vi "PH_PP_CurrentMeas.PC read PA and FR.vi"(0 "i ref in":refnum<vi>, 5 "error in (no error)":errorcluster) -> (14 "i ref out":refnum<vi>, 19 "error out":errorcluster)   [LabVIEW 2014, in "PH_PP_CurrentMeas.lvlib"]
doc: "This VI reads the data from RT client 3 (PA and FR) and sets the GUI elements (if chosen)."
uses:
  PH_PP_CurrentMeas.lvlib
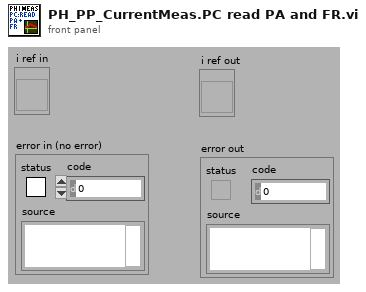
[diagram p1: front panel]
types:
  T1 = typedef "PH_PP_CurrentMeas.lvlib/PH_PP_CurrentMeas.i attribute.ctl" = cluster{"Status":cluster{"GUI Ref Hardware Feedback":refnum<vi>, "Tab Control":refnum<vi>}, "PU 1":cluster{"Instance":string, "Status":T2, "Ref Status ":refnum<vi>, "Data":waveform(dbl)[], "Ref Data":refnum<vi>}, "PU 2":cluster{"Instance":string, "Status":T2, "Ref Status ":refnum<vi>, "Data":waveform(dbl)[], "Ref Data":refnum<vi>}, "PU 3":cluster{"Instance":string, "Status":T2, "Ref Status ":refnum<vi>, "Data":waveform(dbl)[], "Ref Data":refnum<vi>}, "PU 4":cluster{"Instance":string, "Status":T2, "Ref Status ":refnum<vi>, "Data":waveform(dbl)[], "Ref Data":refnum<vi>}, "PU 5":cluster{"Instance":string, "Status":T2, "Ref Status ":refnum<vi>, "Data":waveform(dbl)[], "Ref Data":refnum<vi>}, "FR":cluster{"Instance":string, "Status":T2, "Ref Status ":refnum<vi>, "Data":waveform(dbl)[], "Ref Data":refnum<vi>}, "PA - 19mm 1":cluster{"Instance":string, "Status":T2, "Ref Status ":refnum<vi>}, "PA - 19mm 2":cluster{"Instance":string, "Status":T2, "Ref Status ":refnum<vi>, "no link":bool}, "PA - 45mm":cluster{"Instance":string, "Status":T2, "Ref Status ":refnum<vi>, "no link":bool}, "PA Data":cluster{"Data":waveform(dbl)[], "Ref":refnum<vi>}, "Sequencer":cluster{"Instance":string, "SM State Ref":refnum<vi>}, "Tasks":cluster{"Port":u16, "connection ID":refnum<k5>, "Status":T2, "Ref":refnum<vi>, "Ref Bar":refnum<vi>, "Feedback":cluster{"Received Data Sets":T3[], "Driver Error":errorcluster, "Connection not established":bool, "Error unpacking the data":bool, "No Task defined":bool, "Not triggered yet":bool}, "Data":waveform(dbl)[], "Ref Teststart Task":refnum<vi>}[], "in use":cluster{"MA DP":bool, "FR and PA":bool}, "DAQ Server":string}
  T2 = typedef "PH_StatusHandler.lvlib/PH_StatusHandler.Status.ctl" = i16
  T3 = typedef "PH_PP_CurrentMeas.lvlib/PH_PP_CurrentMeas.CommandCluster.ctl" = cluster{"Command":string, "Data":string, "error out":errorcluster}
  T4 = enum32{"PA 19 DP", "MA 1", "MA 2", "MA 3", "MA 4", "MA 5", "MA FR", "Feedback"}
  T5 = enum32{"PA 19 DP", "MA 1", "MA 2", "MA 3", "MA 4", "MA 5", "MA FR", "Feedback"}[]
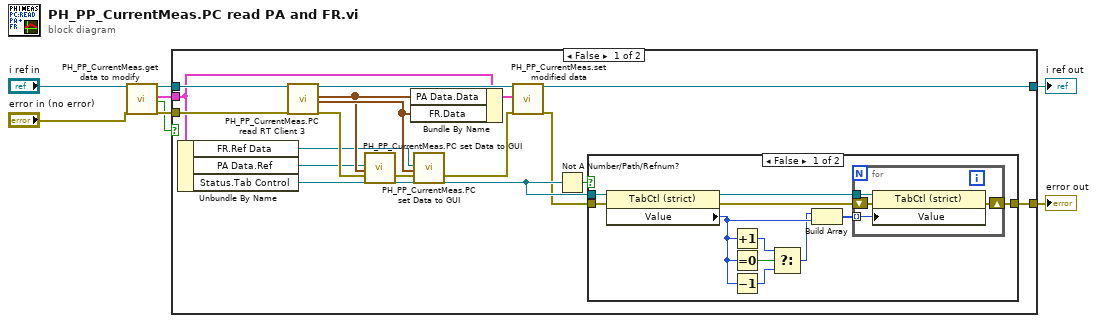
[diagram p0: block diagram]
diagram:
  n1 = call "PH_PP_CurrentMeas.get data to modify.vi"("i ref in"="i ref in", "error in (no error)"="error in (no error)") -> ("i ref out"=w7:refnum<vi>, "i attribute"=w2:T1, "timed out"=w1:bool, "error out"=w8:errorcluster)  [unwired: 14 in]
  n2 = case shown="False" w1 {
    tunnel: w8 -> [w25 w42]
    tunnel: w7 -> [w24 w43]
    tunnel: [w23 w43] -> w4
    tunnel: [w10 w42] -> w3
    tunnel: w2 -> [w20 _]
    frame False {
      n3 = Unbundle By Name(w20) -> ("FR.Ref Data"=w13:refnum<vi>, "PA Data.Ref"=w14:refnum<vi>, "Status.Tab Control"=w12:refnum<vi>)
      n4 = call "PH_PP_CurrentMeas.PC read RT Client 3.vi"("i ref in"=w24, "error in (no error)"=w25) -> ("i ref out"=w22:refnum<vi>, "Data PA"=w15:waveform(dbl)[], "Data MA FR"=w16:waveform(dbl)[], "error out"=w17:errorcluster)  [unwired: 13 in, 1 out]
      n5 = call "PH_PP_CurrentMeas.PC set Data to GUI.vi"("Ref GUI element"=w14, "Data"=w15, "error in (no error)"=w17) -> ("error out"=w19:errorcluster)  [unwired: 16 in]
      n6 = Bundle By Name(cluster=w20, "PA Data.Data"=w15, "FR.Data"=w16) -> (w21:T1)
      n7 = call "PH_PP_CurrentMeas.PC set Data to GUI.vi"("Ref GUI element"=w13, "Data"=w16, "error in (no error)"=w19) -> ("error out"=w18:errorcluster)  [unwired: 16 in]
      n8 = call "PH_PP_CurrentMeas.set modified data.vi"("i ref in"=w22, "i attribute"=w21, "error in (no error)"=w18) -> ("i ref out"=w23:refnum<vi>, "error out"=w11:errorcluster)  [unwired: 15 in]
      n9 = Not A Number/Path/Refnum?(number/path/refnum=w12) -> (NaN/Path/Refnum?=w9:bool)
      n10 = case shown="False" w9 {
        tunnel: [w36 w41] -> w10
        tunnel: w12 -> [w35 _]
        tunnel: w11 -> [w33 w41]
        frame False {
          n11 = property class="TabCtl (strict)"(reference=w35, error in=w33) -> (reference out=w34:refnum<vi>, error out=w32:errorcluster, "Value"=w30:T4)
          n12 = Increment(x=w30) -> (x+1=w28:T4)
          n13 = Equal To 0?(x=w30) -> (x = 0?=w29:bool)
          n14 = Decrement(x=w30) -> (x-1=w27:T4)
          n15 = Select(t=w28, s=w29, f=w27) -> (s? t:f=w26:T4)
          n16 = Build Array(w26, w30) -> (w31:T5)
          n17 = for {
            tunnel: w34 -> [w38]
            shift-right: [w39] -> w36
            shift-left: w32 -> [w40]
            tunnel: w31 -> [w37] mode=indexing
            n18 = property class="TabCtl (strict)"(reference=w38, error in=w40, "Value"=w37) -> (error out=w39:errorcluster)  [unwired: 1 out]
          }
        }
        frame True {
        }
      }
    }
    frame True {
    }
  }
  "error out" <- w3
  "i ref out" <- w4
